vi "Teleop Climb Control.vi"() -> ()   [LabVIEW 2016]
uses:
  Common Code/Gamepads/Button Cluster.ctl
  Robot Global Data.vi
panel:
  in  "Button Cluster":T1
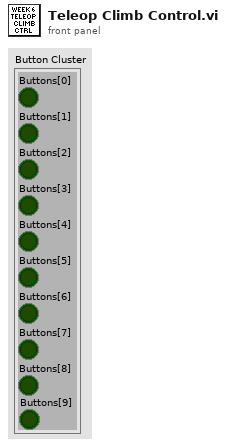
[diagram p1: front panel]
types:
  T1 = typedef "Button Cluster.ctl" = cluster{"Buttons[0]":bool, "Buttons[1]":bool, "Buttons[2]":bool, "Buttons[3]":bool, "Buttons[4]":bool, "Buttons[5]":bool, "Buttons[6]":bool, "Buttons[7]":bool, "Buttons[8]":bool, "Buttons[9]":bool}
  T2 = typedef "Climb Command Cluster.ctl" = cluster{"Power":dbl}
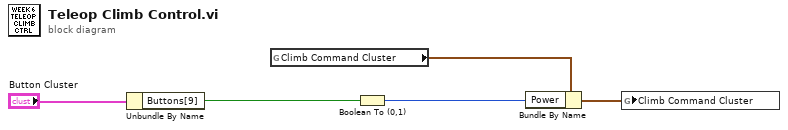
[diagram p0: block diagram]
diagram:
  n1 = Unbundle By Name("Button Cluster") -> ("Buttons[9]"=w2:bool)
  n2 = global read "Robot Global Data.vi" "Climb Command Cluster"() -> (w4:T2)
  n3 = Boolean To (0,1)(Boolean=w2) -> (0, 1=w1:i16)
  n4 = Bundle By Name(cluster=w4, "Power"=w1) -> (w3:T2)
  n5 = global write "Robot Global Data.vi" "Climb Command Cluster"(w3) -> ()
